vi "Untitled 2 (SubVI).vi"(8 "error in (no error)":errorcluster, 9 "Source Code":string, 10 "Script Variable":string, 11 "VISA Refnum in":refnum<visa-resource-name>) -> (0 "error out":errorcluster, 3 "VISA Refnum out":refnum<visa-resource-name>)   [LabVIEW 2020, in "Keithley 2600 Series.lvlib"]
uses:
  <instrlib>/Keithley 2600 Series/Keithley 2600 Series.lvlib
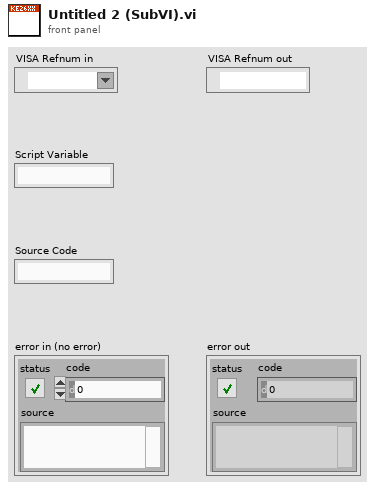
[diagram p1: front panel]
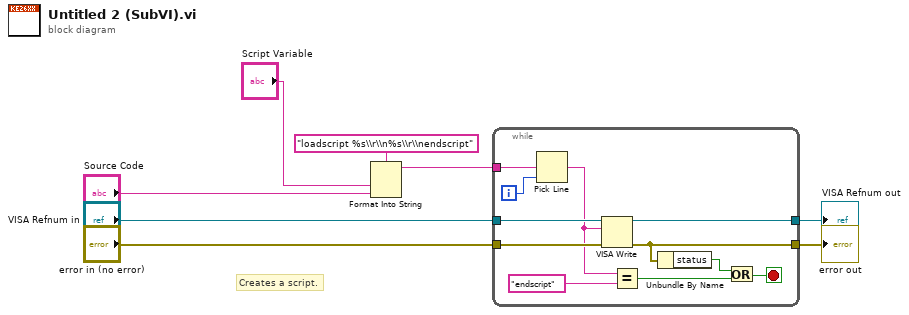
[diagram p0: block diagram]
diagram:
  # "Creates a script."
  n1 = Format Into String(format string="loadscript %s\\r\\n%s\\r\\nendscript", "Script Variable", "Source Code") -> (resulting string=w5:string)  [unwired: 2 in, 1 out]
  n2 = while {
    tunnel: "VISA Refnum in" -> [w19]
    tunnel: "error in (no error)" -> [w18]
    tunnel: [w17] -> w6
    tunnel: [w14] -> w7
    tunnel: w5 -> [w16]
    i -> [w15]
    stop <- w12 stop-if-true
    n3 = Pick Line(multi-line string=w16, line index=w15) -> (output string=w11:string)  [unwired: 1 in]
    n4 = VISA Write(VISA resource name=w19, write buffer=w11, error in (no error)=w18) -> (VISA resource name out=w17:refnum<visa-resource-name>, error out=w14:errorcluster)  [unwired: 1 out]
    n5 = Equal?(x=w11, y="endscript") -> (x = y?=w9:bool)
    n6 = Unbundle By Name(w14) -> ("status"=w13:bool)
    n7 = Or(x=w13, y=w9) -> (x .or. y?=w12:bool)
  }
  "error out" <- w7
  "VISA Refnum out" <- w6
